vi "Update.vi"(8 "Error In":errorcluster, 10 "CommunicationModule":refnum<class "CommunicationModule.lvclass">, 11 "reference in":refnum<class "Controller.lvclass">) -> (0 "Error Out":errorcluster, 3 "reference out":refnum<class "Controller.lvclass">)   [LabVIEW 2024, in "Controller.lvclass"]
uses:
  Controller.lvclass
  Controller.lvclass/Controller.ctl
  CommunicationModule/CommunicationModule.lvclass
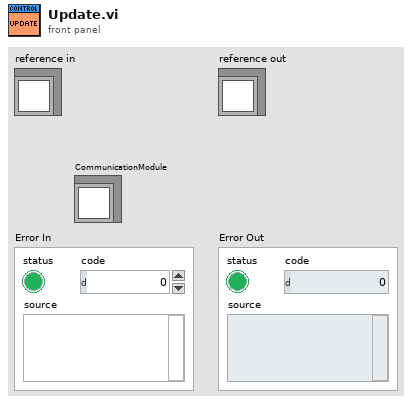
[diagram p1: front panel]
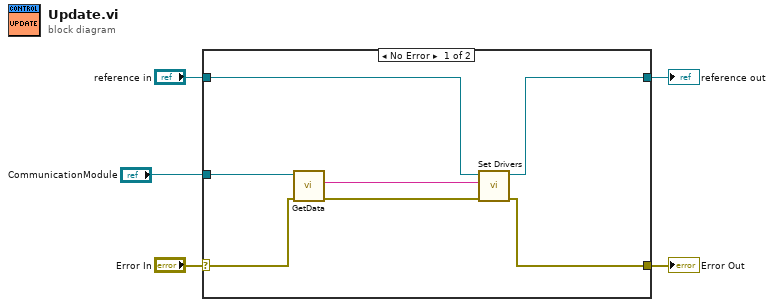
[diagram p0: block diagram]
diagram:
  n1 = case shown="No Error" "Error In" {
    selector: "Error In" -> [w11 w14]
    tunnel: [w7 w14] -> w4
    tunnel: [w9 w13] -> w2
    tunnel: "reference in" -> [w10 w13]
    tunnel: "CommunicationModule" -> [w12 _]
    frame No Error {
      n2 = call-dynamic "GetData.vi"("Error In"=w11, "reference in"=w12) -> ("Error Out"=w8:errorcluster, "Data"=w6:string)  [unwired: 7 in, 1 out]
      n3 = call-dynamic "Set Drivers.vi"("Error In"=w8, "Data"=w6, "reference in"=w10) -> ("Error Out"=w7:errorcluster, "reference out"=w9:refnum<class "Controller.lvclass">)  [unwired: 7 in]
    }
    frame Error {
    }
  }
  "Error Out" <- w4
  "reference out" <- w2
